vi "DS18x20 - top level.vi"() -> ()   [LabVIEW 2013]
uses:
  Type Defs/ROM Commands.ctl
  Type Defs/Master Function Commands.ctl
panel:
  out "Convert Time (usec)":u32
  out "Supply Mode":bool
  in  "Reset Delay (ms)":u32=100
  in  "stop":bool
  in  "Execute":bool
  out "Scratchpad Data":u8[](array[numeric]) format="%.0x"
  in  "Master Function Command":T1
  out "ROM Data":u8[](array[numeric]) format="%.0x"
  in  "ROM Command":T2=enum."Skip ROM Command"
  out "error out":errorcluster
  in  "error in":errorcluster
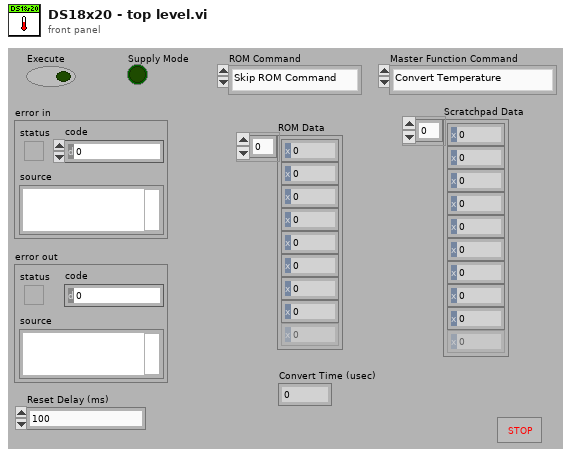
[diagram p1: front panel]
types:
  T1 = typedef "Master Function Commands.ctl" = enum16{"Convert Temperature", "Read Scratchpad", "Read Power Supply"}
  T2 = typedef "ROM Commands.ctl" = enum16{"Read ROM", "Skip ROM Command"}
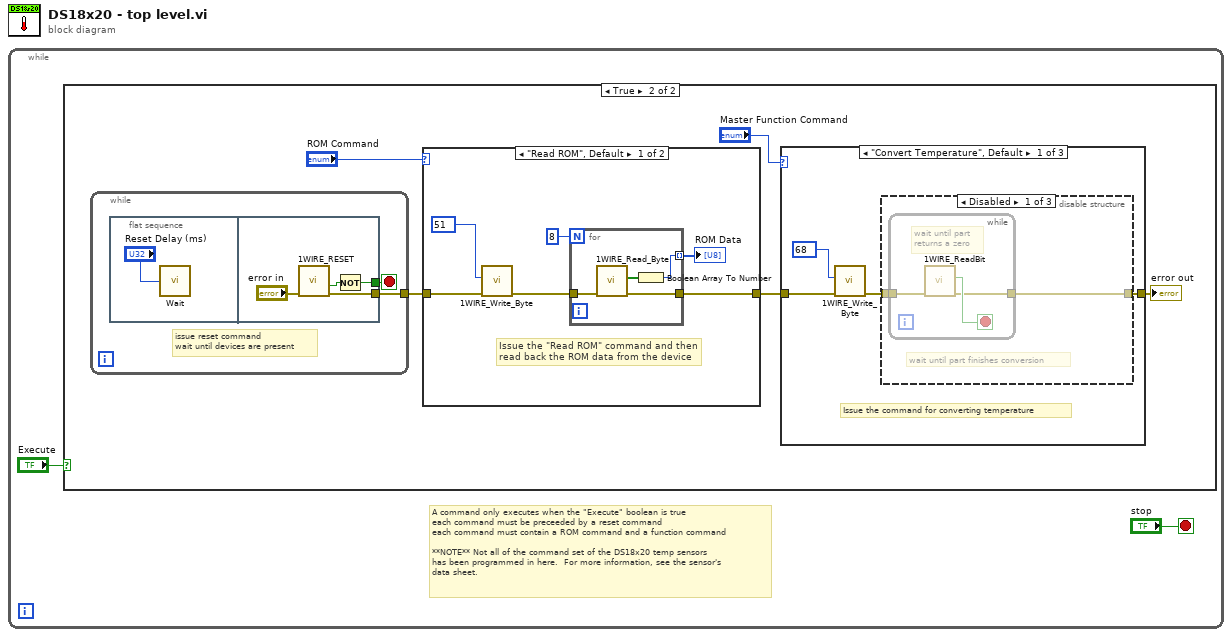
[diagram p0: block diagram]
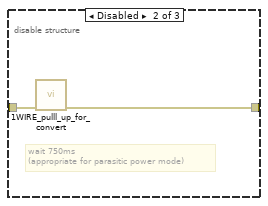
[diagram p3: hidden frame]
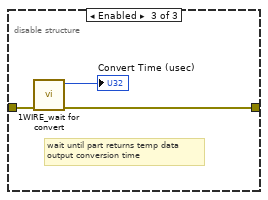
[diagram p4: hidden frame]
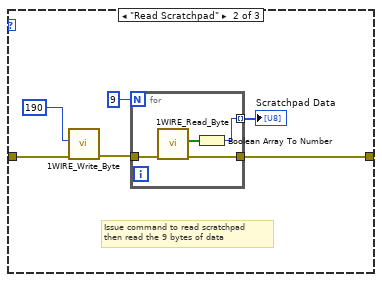
[diagram p5: hidden frame]
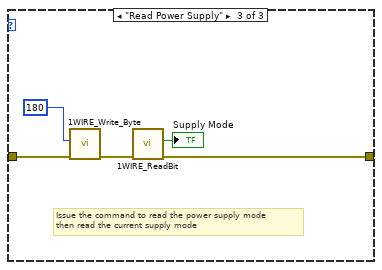
[diagram p6: hidden frame]
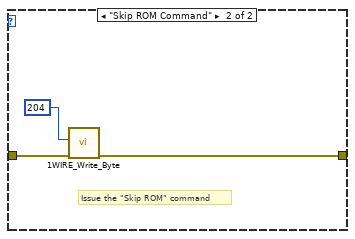
[diagram p7: hidden frame]
diagram:
  n1 = while {
    stop <- "stop" stop-if-true
    # "A command only executes when the \"Execute\" boolean is true\neach command must be preceeded by a reset command\neach command must contain a ROM command and a function command\n\n**NOTE** Not all of the command set of the DS18x20 temp sensors\nhas been programmed in here.  For more information, see the sensor's\ndata sheet."
    n2 = case shown="True" "Execute" {
      frame False {
      }
      frame True {
        n3 = while {
          tunnel: [w50] -> w5
          stop <- w51 stop-if-true
          # "issue reset command\nwait until devices are present"
          n4 = flat-sequence {
            tunnel: [w55] -> w51
            tunnel: [w54] -> w50
            frame #0 {
              n5 = call "Wait"("Count(mSec)"="Reset Delay (ms)") -> ()  [unwired: 1 out]
            }
            frame #1 {
              n6 = call "1WIRE_RESET.vi"("error in"="error in") -> ("error out"=w54:errorcluster, "0 = Device Present / 1=no"=w53:bool)  [unwired: 9 in]
              n7 = Not(x=w53) -> (.not. x?=w55:bool)
            }
          }
        }
        n8 = case shown="\"Read ROM\", Default" "ROM Command" {
          tunnel: w5 -> [w40 w49]
          tunnel: [w38 w48] -> w4
          frame "Read ROM", Default {
            # "Issue the \"Read ROM\" command and then\nread back the ROM data from the device"
            n9 = call "1WIRE_Write_Byte.vi"("error in"=w40, "Tx data"=u8 51 ("Tx data 2")) -> ("error out"=w42:errorcluster)  [unwired: 8 in, 1 out]
            n10 = for {
              N: 8 -> [_]
              tunnel: w42 -> [w46]
              tunnel: [w45] -> w38
              tunnel: [w43] -> w39 mode=indexing
              n11 = call "1WIRE_Read_Byte.vi"("error in"=w46) -> ("error out"=w45:errorcluster, "Array"=w44:bool[])  [unwired: 9 in]
              n12 = Boolean Array To Number(Boolean array=w44) -> (number=w43:u8)
            }
            "ROM Data" <- w39
          }
          frame "Skip ROM Command" {
            # "Issue the \"Skip ROM\" command"
            n13 = call "1WIRE_Write_Byte.vi"("error in"=w49, "Tx data"=u8 204) -> ("error out"=w48:errorcluster)  [unwired: 8 in, 1 out]
          }
        }
        n14 = case shown="\"Convert Temperature\", Default" "Master Function Command" {
          tunnel: w4 -> [w11 w24 w35]
          tunnel: [w9 w23 w33] -> w6
          frame "Convert Temperature", Default {
            # "Issue the command for converting temperature"
            n15 = call "1WIRE_Write_Byte.vi"("error in"=w11, "Tx data"=u8 68 ("Tx data 2")) -> ("error out"=w10:errorcluster)  [unwired: 8 in, 1 out]
            n16 = disable-structure shown="Disabled" {
              disable-tunnel: w10 -> [w13 w18 w21]
              disable-tunnel: [w12 w17 w20] -> w9
              frame Disabled {
                # "wait until part finishes conversion"
                n17 = while {
                  tunnel: w13 -> [w16]
                  tunnel: [w14] -> w12
                  stop <- w15 stop-if-true
                  # "wait until part\nreturns a zero"
                  n18 = call "1WIRE_ReadBit.vi"("error in"=w16) -> ("error out"=w14:errorcluster, "Bit Read"=w15:bool)  [unwired: 9 in]
                }
              }
              frame Disabled {
                # "wait 750ms\n(appropriate for parasitic power mode)"
                n19 = call "1WIRE_pulll_up_for_convert.vi"("error in"=w18) -> ("error out"=w17:errorcluster)  [unwired: 10 in]
              }
              frame Enabled {
                # "wait until part returns temp data\noutput conversion time"
                n20 = call "1WIRE_wait for convert.vi"("error in"=w21) -> ("error out"=w20:errorcluster, "Convert Time (usec)"=→"Convert Time (usec)":u32)  [unwired: 9 in]
              }
            }
          }
          frame "Read Scratchpad" {
            # "Issue command to read scratchpad\nthen read the 9 bytes of data"
            n21 = call "1WIRE_Write_Byte.vi"("error in"=w24, "Tx data"=u8 190 ("Tx data 2")) -> ("error out"=w25:errorcluster)  [unwired: 8 in, 1 out]
            n22 = for {
              N: 9 -> [_]
              tunnel: w25 -> [w31]
              tunnel: [w30] -> w23
              tunnel: [w28] -> w27 mode=indexing
              n23 = call "1WIRE_Read_Byte.vi"("error in"=w31) -> ("error out"=w30:errorcluster, "Array"=w29:bool[])  [unwired: 9 in]
              n24 = Boolean Array To Number(Boolean array=w29) -> (number=w28:u8)
            }
            "Scratchpad Data" <- w27
          }
          frame "Read Power Supply" {
            # "Issue the command to read the power supply mode\nthen read the current supply mode"
            n25 = call "1WIRE_Write_Byte.vi"("error in"=w35, "Tx data"=u8 180 ("Tx data 2")) -> ("error out"=w34:errorcluster)  [unwired: 8 in, 1 out]
            n26 = call "1WIRE_ReadBit.vi"("error in"=w34) -> ("error out"=w33:errorcluster, "Bit Read"=→"Supply Mode":bool)  [unwired: 9 in]
          }
        }
        "error out" <- w6
      }
    }
  }
